vi "Node - Read Local Channels Table.vi"(8 "error in (no error)":errorcluster, 11 "Compiled.Settings In":T1) -> (0 "error out":errorcluster, 3 "Compiled.Settings Out":T1)   [LabVIEW 2016, in "PXImc Custom Device System Explorer.lvlib"]
uses:
  PXImc Custom Device System Explorer.lvlib
  Shared/Compiled.Settings.ctl
  PXImc Router/Controls/Target Type.ctl
  PXImc Router/Controls/Router - Configuration.ctl
  PXImc Router/Controls/Router/Node Block R-W Properties.ctl
  PXImc Router/Controls/Router/Block Properties.ctl
  PXImc Router/Controls/Router/Router - PXImc Properties.ctl
  PXImc Router/Controls/Router/Router - PXImc Card Properties.ctl
  PXImc Router/Controls/Node Data.ctl
  PXImc Router/Controls/Node/Node - PXImc Parameters.ctl
  PXImc Router/Controls/Node/Node - Writer Data.ctl
  PXImc Router/Controls/Node/Node Ch Properties.ctl
  PXImc Router/Controls/Data Type.ctl
  PXImc Router/Controls/Node/Node - Readers Data.ctl
  PXImc Router/Controls/Node/Node - Reader Data.ctl
  <vilib>/Utility/file.llb/Read Delimited Spreadsheet (string).vi
  PXImc Router/PXImc Router.lvlib
  Shared/PXImc Custom Device Shared.lvlib
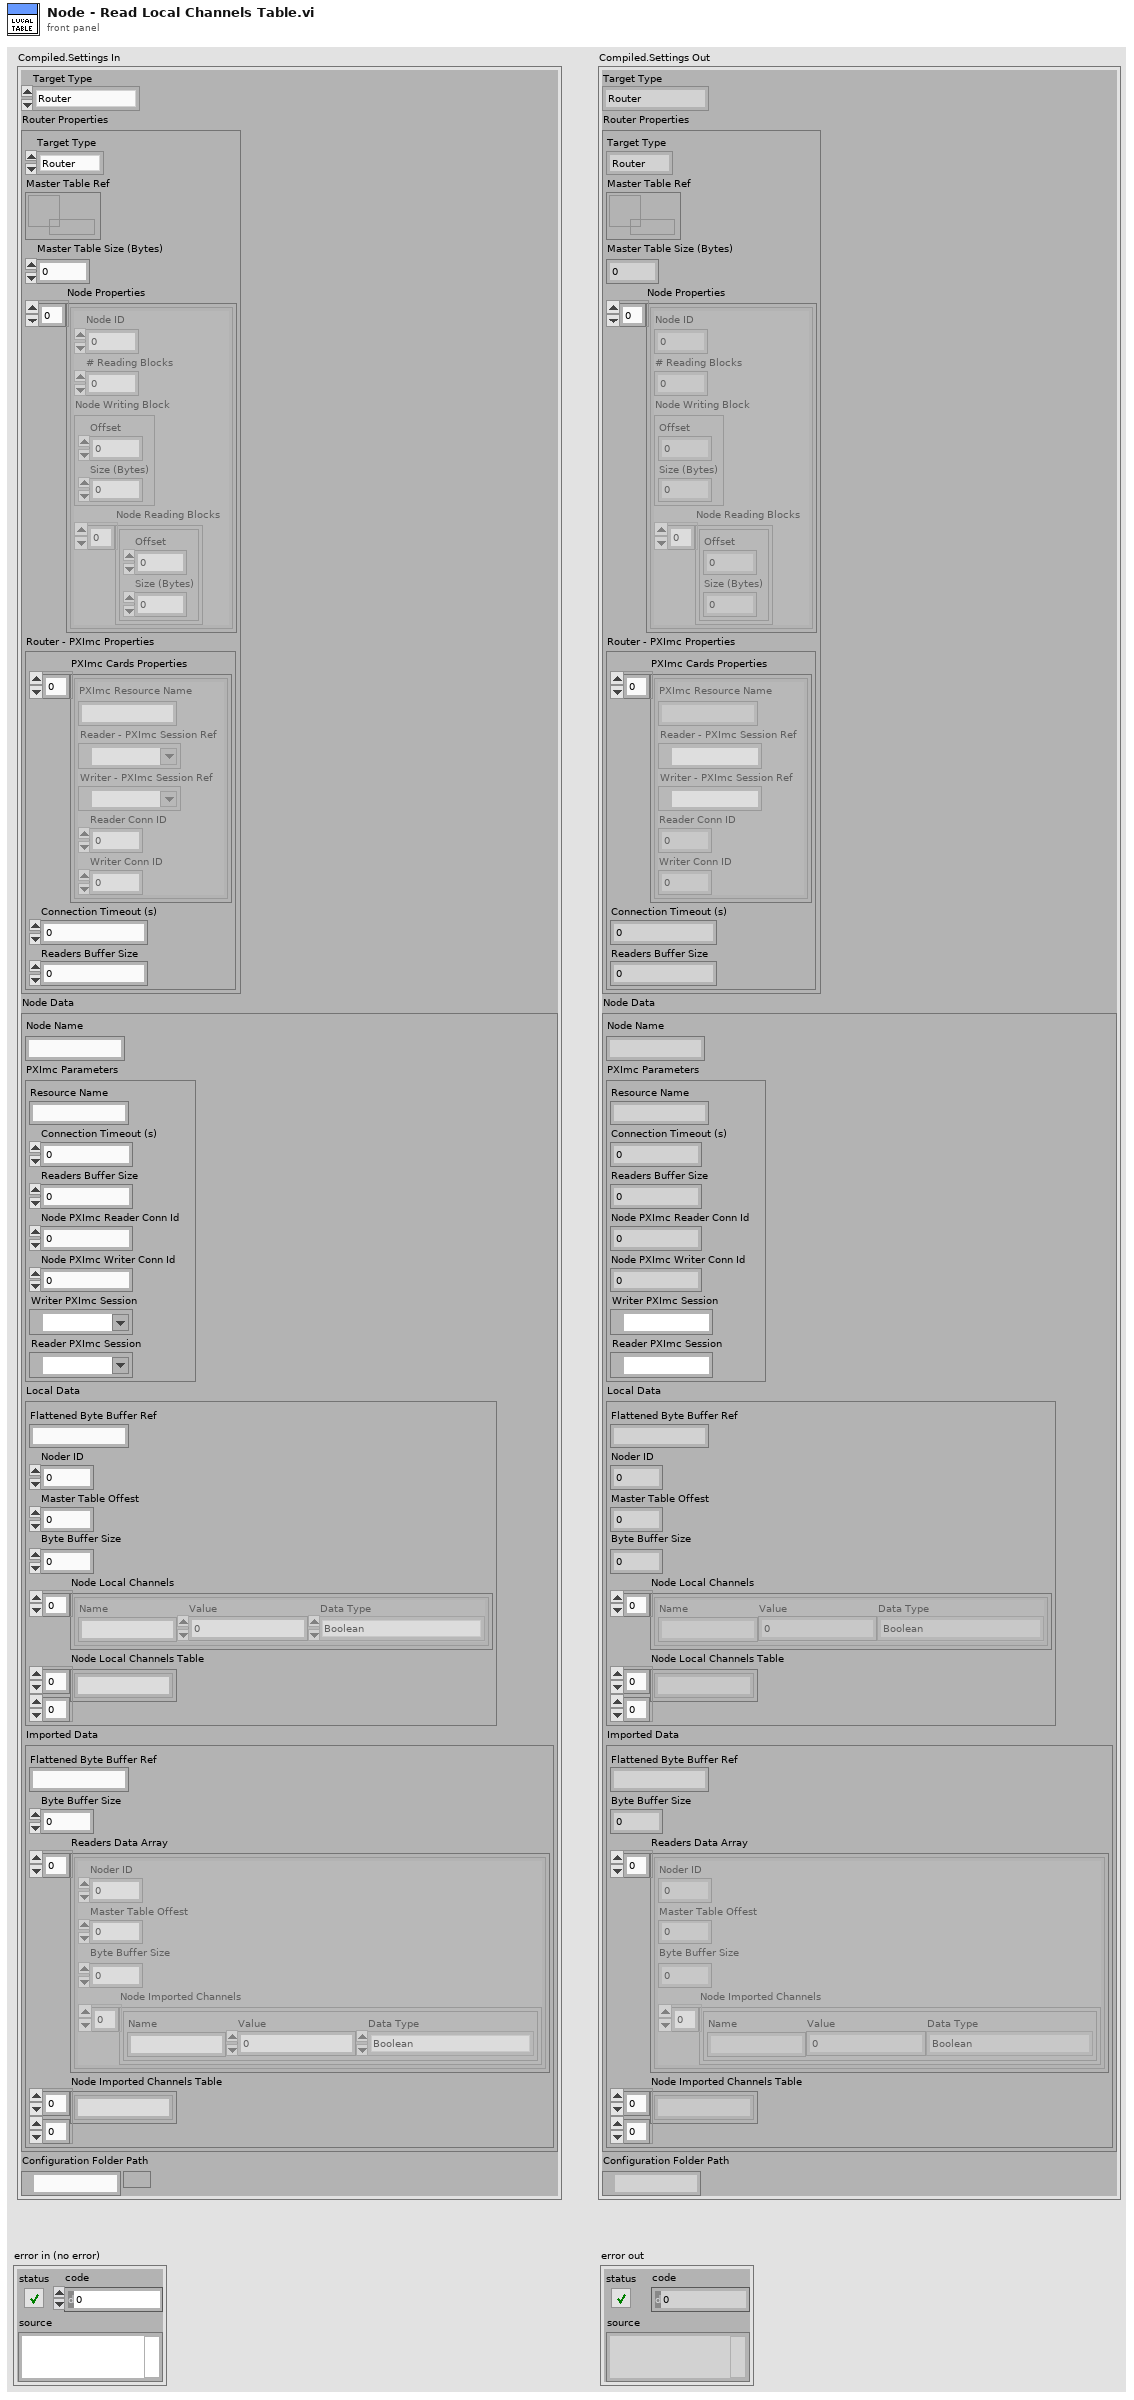
[diagram p1: front panel]
types:
  T1 = typedef "PXImc Custom Device Shared.lvlib/Compiled.Settings.ctl" = cluster{"Target Type":T2, "Router Properties":T3, "Node Data":T8, "Configuration Folder Path":path}
  T2 = typedef "PXImc Router.lvlib/Target Type.ctl" = enum16{"Router", "Node"}
  T3 = typedef "PXImc Router.lvlib/Router - Configuration.ctl" = cluster{"Target Type":T2, "Master Table Ref":refnum<data-value>, "Master Table Size (Bytes)":u32, "Node Properties":T4[], "Router - PXImc Properties":T6}
  T4 = typedef "PXImc Router.lvlib/Node Block R-W Properties.ctl" = cluster{"Node ID":u32, "# Reading Blocks":u32, "Node Writing Block":T5, "Node Reading Blocks":T5[]}
  T5 = typedef "PXImc Router.lvlib/Block Properties.ctl" = cluster{"Offset":u32, "Size (Bytes)":u32}
  T6 = typedef "PXImc Router.lvlib/Router - PXImc Properties.ctl" = cluster{"PXImc Cards Properties":T7[], "Connection Timeout (s)":dbl, "Readers Buffer Size":u64}
  T7 = typedef "PXImc Router.lvlib/Router - PXImc Card Properties.ctl" = cluster{"PXImc Resource Name":string, "Reader - PXImc Session Ref":refnum<k21>, "Writer - PXImc Session Ref":refnum<k21>, "Reader Conn ID":u16, "Writer Conn ID":u16}
  T8 = typedef "PXImc Router.lvlib/Node Data.ctl" = cluster{"Node Name":string, "PXImc Parameters":T9, "Local Data":T10, "Imported Data":T13}
  T9 = typedef "PXImc Router.lvlib/Node - PXImc Parameters.ctl" = cluster{"Resource Name":string, "Connection Timeout (s)":dbl, "Readers Buffer Size":u64, "Node PXImc Reader Conn Id":u16, "Node PXImc Writer Conn Id":u16, "Writer PXImc Session":refnum<k21>, "Reader PXImc Session":refnum<k21>}
  T10 = typedef "PXImc Router.lvlib/Node - Writer Data.ctl" = cluster{"Flattened Byte Buffer Ref":string, "Noder ID":u32, "Master Table Offest":u32, "Byte Buffer Size":u32, "Node Local Channels":T11[], "Node Local Channels Table":string[][]}
  T11 = typedef "PXImc Router.lvlib/Node Ch Properties.ctl" = cluster{"Name":string, "Value":dbl, "Data Type":T12}
  T12 = typedef "PXImc Router.lvlib/Data Type.ctl" = enum16{"Boolean", "SGL", "DBL", "I8", "I16", "I32", "I64", "U8", "U16", "U32", "U64"}
  T13 = typedef "PXImc Router.lvlib/Node - Readers Data.ctl" = cluster{"Flattened Byte Buffer Ref":string, "Byte Buffer Size":u64, "Readers Data Array":T14[], "Node Imported Channels Table":string[][]}
  T14 = typedef "PXImc Router.lvlib/Node - Reader Data.ctl" = cluster{"Noder ID":u32, "Master Table Offest":u32, "Byte Buffer Size":u64, "Node Imported Channels":T11[]}
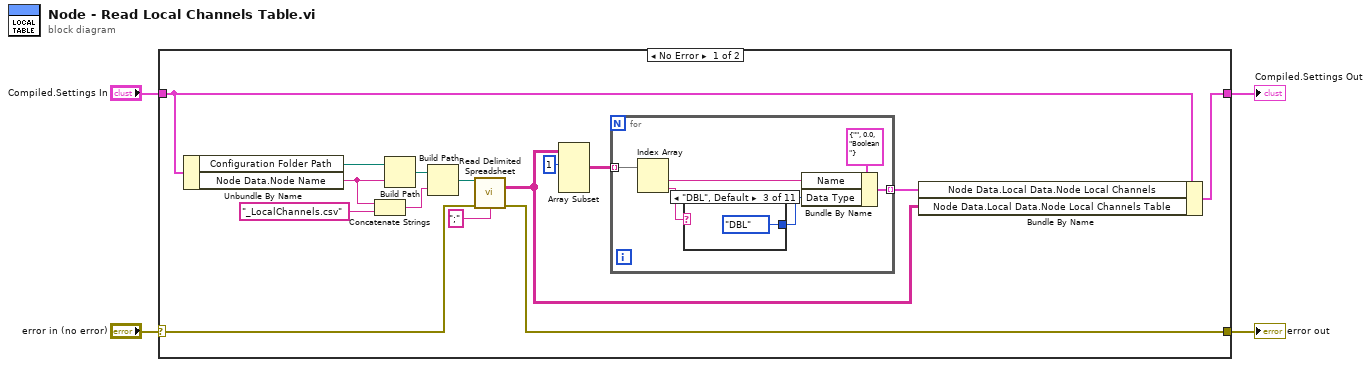
[diagram p0: block diagram]
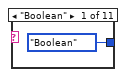
[diagram p2: hidden frame]
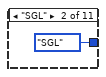
[diagram p3: hidden frame]
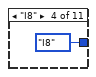
[diagram p4: hidden frame]
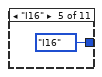
[diagram p5: hidden frame]
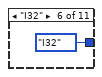
[diagram p6: hidden frame]
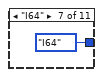
[diagram p7: hidden frame]
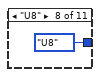
[diagram p8: hidden frame]
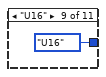
[diagram p9: hidden frame]
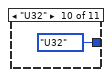
[diagram p10: hidden frame]
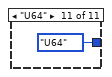
[diagram p11: hidden frame]
diagram:
  n1 = case shown="No Error" "error in (no error)" {
    selector: "error in (no error)" -> [w9 w37]
    tunnel: "Compiled.Settings In" -> [w15 w38]
    tunnel: [w16 w38] -> w3
    tunnel: [w8 w37] -> w1
    frame No Error {
      n2 = Unbundle By Name(w15) -> ("Configuration Folder Path"=w14:path, "Node Data.Node Name"=w7:string)
      n3 = Concatenate Strings(w7, "_LocalChannels.csv" ("name or relative path")) -> (w12:string)
      n4 = Build Path(base path=w14, name or relative path=w7) -> (appended path=w19:path)
      n5 = Build Path(base path=w19, name or relative path=w12) -> (appended path=w18:path)
      n6 = call-poly <vilib>:"Read Delimited Spreadsheet.vi"("file path (dialog if empty)"=w18, "error in (no error)"=w9, "delimiter (\\t)"=";" ("delimiter (\\t)")) -> ("all rows"=w5:string[][], "error out"=w8:errorcluster)  [unwired: 7 in, 4 out]
      n7 = Array Subset(array=w5, index (row)=1 ("index")) -> (w6:string[][])  [unwired: 3 in]
      n8 = for {
        tunnel: [w25] -> w10 mode=indexing
        tunnel: w6 -> [w24] mode=indexing
        n9 = Index Array(array=w24) -> (element #1=w21:string, element #2=w20:string)  [unwired: 2 in]
        n10 = case shown="\"DBL\", Default" w20 {
          tunnel: [Data_Type."Boolean" ("Data Type") Data_Type."SGL" ("Data Type") Data_Type."DBL" ("Data Type") Data_Type."I8" ("Data Type") Data_Type."I16" ("Data Type") Data_Type."I32" ("Data Type") Data_Type."I64" ("Data Type") Data_Type."U8" ("Data Type") Data_Type."U16" ("Data Type") Data_Type."U32" ("Data Type") Data_Type."U64" ("Data Type")] -> w23
          frame "Boolean" {
          }
          frame "SGL" {
          }
          frame "DBL", Default {
          }
          frame "I8" {
          }
          frame "I16" {
          }
          frame "I32" {
          }
          frame "I64" {
          }
          frame "U8" {
          }
          frame "U16" {
          }
          frame "U32" {
          }
          frame "U64" {
          }
        }
        n11 = Bundle By Name(cluster=T11 {"Name"="", "Value"=0.0, "Data Type"=enum."Boolean"} ("Node Ch Properties"), "Name"=w21, "Data Type"=w23) -> (w25:T11)
      }
      n12 = Bundle By Name(cluster=w15, "Node Data.Local Data.Node Local Channels"=w10, "Node Data.Local Data.Node Local Channels Table"=w5) -> (w16:T1)
    }
    frame Error {
    }
  }
  "Compiled.Settings Out" <- w3
  "error out" <- w1
